vi "OUT-READ(subvi).vi"(8 "error in (no error)":errorcluster, 11 "ARRAY IN":string[](array[string])) -> (0 "error out":errorcluster, 2 "Salidas":bool[](array[boolean]))   [LabVIEW 2014, in "CAP-USB.lvlib"]
doc: "VI encargado de leer el valor de las entradas que envia el \nCAP-USB"
uses:
  CAP-USB.lvlib
  0-Nivel/Enum DI-Reader.ctl
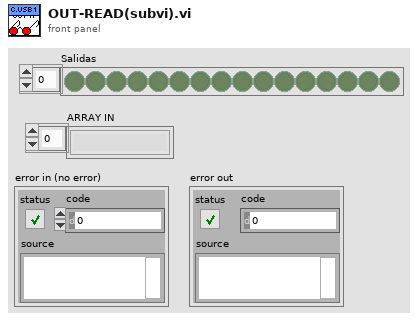
[diagram p1: front panel]
types:
  T1 = typedef "CAP-USB.lvlib/Enum DI-Reader.ctl" = enum16{"IDLE", "Detect XX", "Detect YY", "Valor", ""}
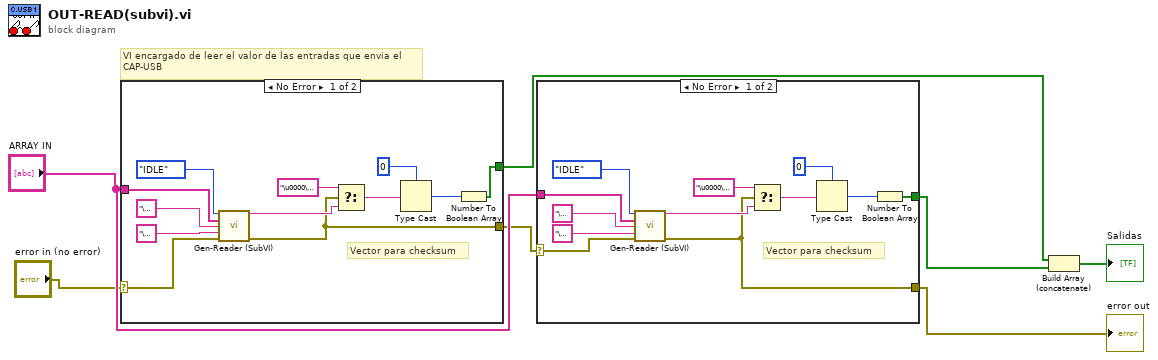
[diagram p0: block diagram]
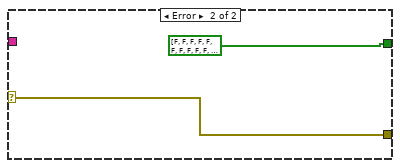
[diagram p2: hidden frame]
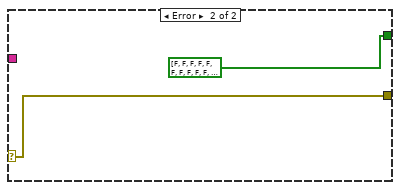
[diagram p3: hidden frame]
diagram:
  # "VI encargado de leer el valor de las entradas que envia el \nCAP-USB"
  n1 = case shown="No Error" "error in (no error)" {
    selector: "error in (no error)" -> [w16 w20]
    tunnel: [w17 bool[] [FALSE, FALSE, FALSE, FALSE, FALSE, FALSE, FALSE, FALSE, FALSE, FALSE, FALSE, FALSE, FALSE, FALSE, FALSE, FALSE] ("Boolean array")] -> w7
    tunnel: "ARRAY IN" -> [w11 _]
    tunnel: [w8 w20] -> w2
    frame No Error {
      # "Vector para checksum"
      n2 = call "Gen-Reader (SubVI).vi"("Enum"=Enum_DI-Reader."IDLE", "ARRAY IN"=w11, "XX"="\u0003", "YY"="\u0001", "error in (no error)"=w16) -> ("read buffer"=w19:string, "error out"=w8:errorcluster)  [unwired: 8 in, 1 out]
      n3 = Select(t="\u0000\u0000", s=w8, f=w19) -> (s? t:f=w15:string)
      n4 = Type Cast(type=u8 0 ("default (0 U32)"), x=w15) -> (*(type *) &x=w14:u8)
      n5 = Number To Boolean Array(number=w14) -> (Boolean array=w17:bool[])
    }
    frame Error {
    }
  }
  n6 = case shown="No Error" w2 {
    selector: w2 -> [w29 w35]
    tunnel: [w31 w35] -> w1
    tunnel: [w30 bool[] [FALSE, FALSE, FALSE, FALSE, FALSE, FALSE, FALSE, FALSE, FALSE, FALSE, FALSE, FALSE, FALSE, FALSE, FALSE, FALSE] ("Boolean array")] -> w6
    tunnel: "ARRAY IN" -> [w24 _]
    frame No Error {
      # "Vector para checksum"
      n7 = call "Gen-Reader (SubVI).vi"("Enum"=Enum_DI-Reader."IDLE", "ARRAY IN"=w24, "XX"="\u0003", "YY"="\u0005", "error in (no error)"=w29) -> ("read buffer"=w33:string, "error out"=w31:errorcluster)  [unwired: 8 in, 1 out]
      n8 = Select(t="\u0000\u0000", s=w31, f=w33) -> (s? t:f=w28:string)
      n9 = Type Cast(type=u8 0 ("default (0 U32)"), x=w28) -> (*(type *) &x=w27:u8)
      n10 = Number To Boolean Array(number=w27) -> (Boolean array=w30:bool[])
    }
    frame Error {
    }
  }
  "error out" <- w1
  n11 = Build Array (concatenate)(w7, w6) -> (→"Salidas":bool[])
